vi "CreateTask.vi"(8 "error in":errorcluster, 10 "data":T1={"IMAQDeviceName"="", "LocalSavingPath"=path "", "Save"=enum."off", "Timeout"={"Value"=0.0, "Min"=0.0, "Max"=0.0, "StepSize"=0.0, "Tolerance"=0.0, "ValueActual"=0.0}, "Min Temperature"={"Value"=0.0, "Min"=18.0, "Max"=50.0, "StepSize"=0.0, "Tolerance"=0.0, "ValueActual"=0.0}, "aiChannel"="", "CJC_Value"={"Value"=0.0, "Min"=0.0, "Max"=0.0, "StepSize"=0.0, "Tolerance"=0.0, "ValueActual"=0.0}, "Thermocouple Type"=enum."E", "units"=enum."From Custom Scale", "CJC Source"=enum."Channel", "CJC Channel"="", "Simulation"=enum."off", "Max Temperature"={"Value"=0.0, "Min"=18.0, "Max"=50.0, "StepSize"=0.0, "Tolerance"=0.0, "ValueActual"=0.0}}, 11 "NI-TC-01 in":refnum<class "NI-TC-01.lvclass">) -> (0 "error out":errorcluster, 2 "data Out":T1={"IMAQDeviceName"="", "LocalSavingPath"=path "", "Save"=enum."off", "Timeout"={"Value"=0.0, "Min"=0.0, "Max"=0.0, "StepSize"=0.0, "Tolerance"=0.0, "ValueActual"=0.0}, "Min Temperature"={"Value"=0.0, "Min"=18.0, "Max"=50.0, "StepSize"=0.0, "Tolerance"=0.0, "ValueActual"=0.0}, "aiChannel"="", "CJC_Value"={"Value"=0.0, "Min"=0.0, "Max"=0.0, "StepSize"=0.0, "Tolerance"=0.0, "ValueActual"=0.0}, "Thermocouple Type"=enum."E", "units"=enum."From Custom Scale", "CJC Source"=enum."Channel", "CJC Channel"="", "Simulation"=enum."off", "Max Temperature"={"Value"=0.0, "Min"=18.0, "Max"=50.0, "StepSize"=0.0, "Tolerance"=0.0, "ValueActual"=0.0}}, 3 "NI-TC-01 out":refnum<class "NI-TC-01.lvclass">)   [LabVIEW 2013, in "NI-TC-01.lvclass"]
uses:
  NI-TC-01.lvclass
  settings_TypDef.ctl
  shared/OnOffTypeDef.ctl
  shared/numericVariable_TypeDef.ctl
  NI-TC-01.lvclass/NI-TC-01.ctl
  <vilib>/DAQmx/create/channels.llb/DAQmx Create Channel (AI-Temperature-Thermocouple).vi
  BaseDriver/BaseDriver.lvclass
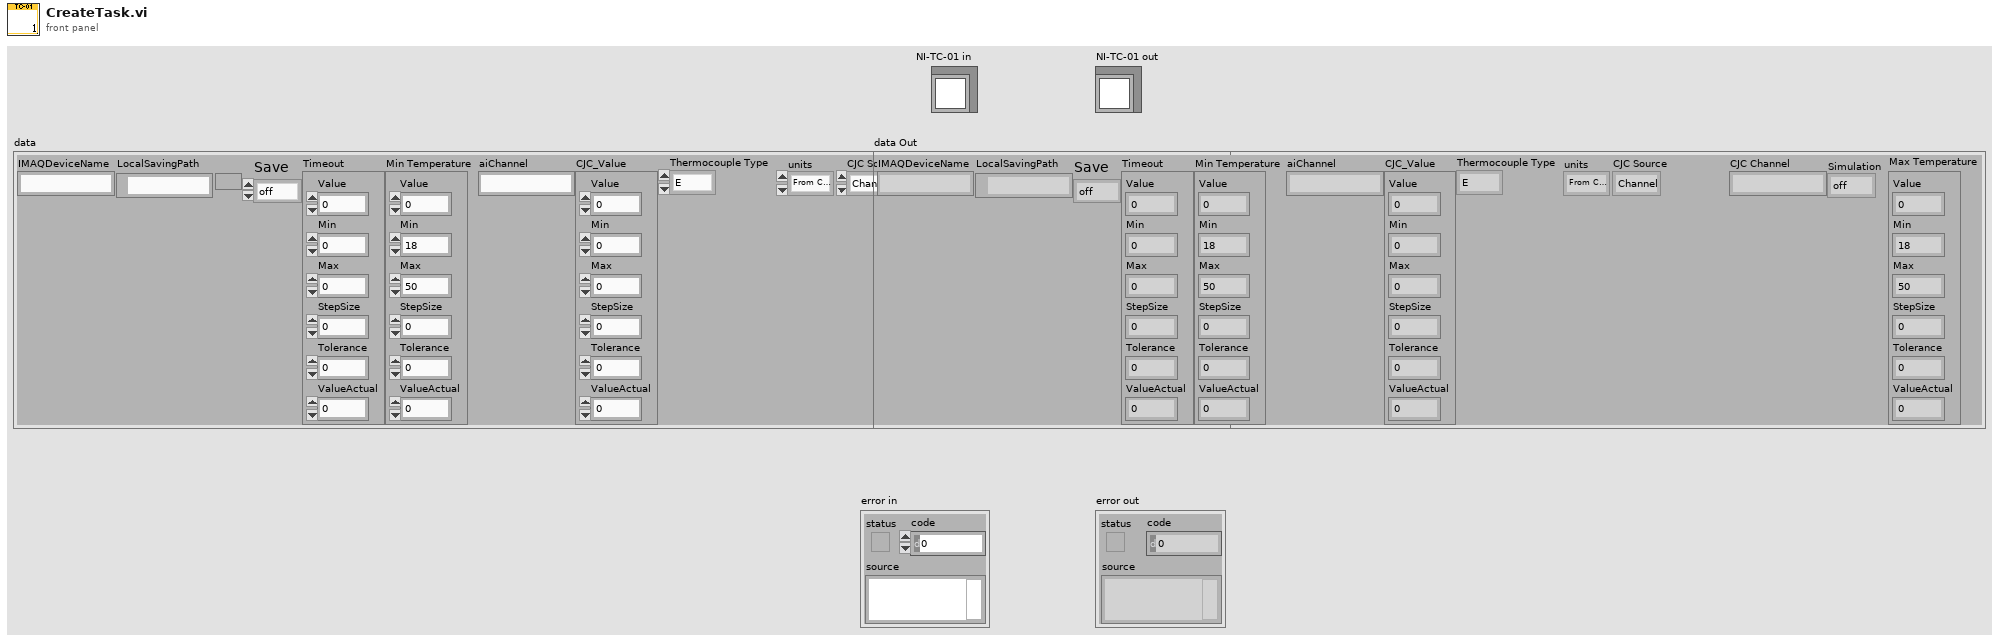
[diagram p1: front panel]
types:
  T1 = typedef "NI-TC-01.lvclass/settings_TypDef.ctl" = cluster{"IMAQDeviceName":string, "LocalSavingPath":path, "Save":T2, "Timeout":T3, "Min Temperature":T3, "aiChannel":string, "CJC_Value":T3, "Thermocouple Type":enum16{"J", "K", "N", "R", "S", "T", "B", "E"}, "units":enum16{"Deg C", "Deg F", "Kelvins", "Deg R", "From Custom Scale"}, "CJC Source":enum16{"Built-In", "Constant Value", "Channel"}, "CJC Channel":string, "Simulation":T2, "Max Temperature":T3}
  T2 = typedef "OnOffTypeDef.ctl" = enum16{"off", "on"}
  T3 = typedef "BaseDriver.lvclass/numericVariable_TypeDef.ctl" = cluster{"Value":dbl, "Min":dbl, "Max":dbl, "StepSize":dbl, "Tolerance":dbl, "ValueActual":dbl}
  T4 = enum16{"Deg C", "Deg F", "Kelvins", "Deg R", "From Custom Scale"}
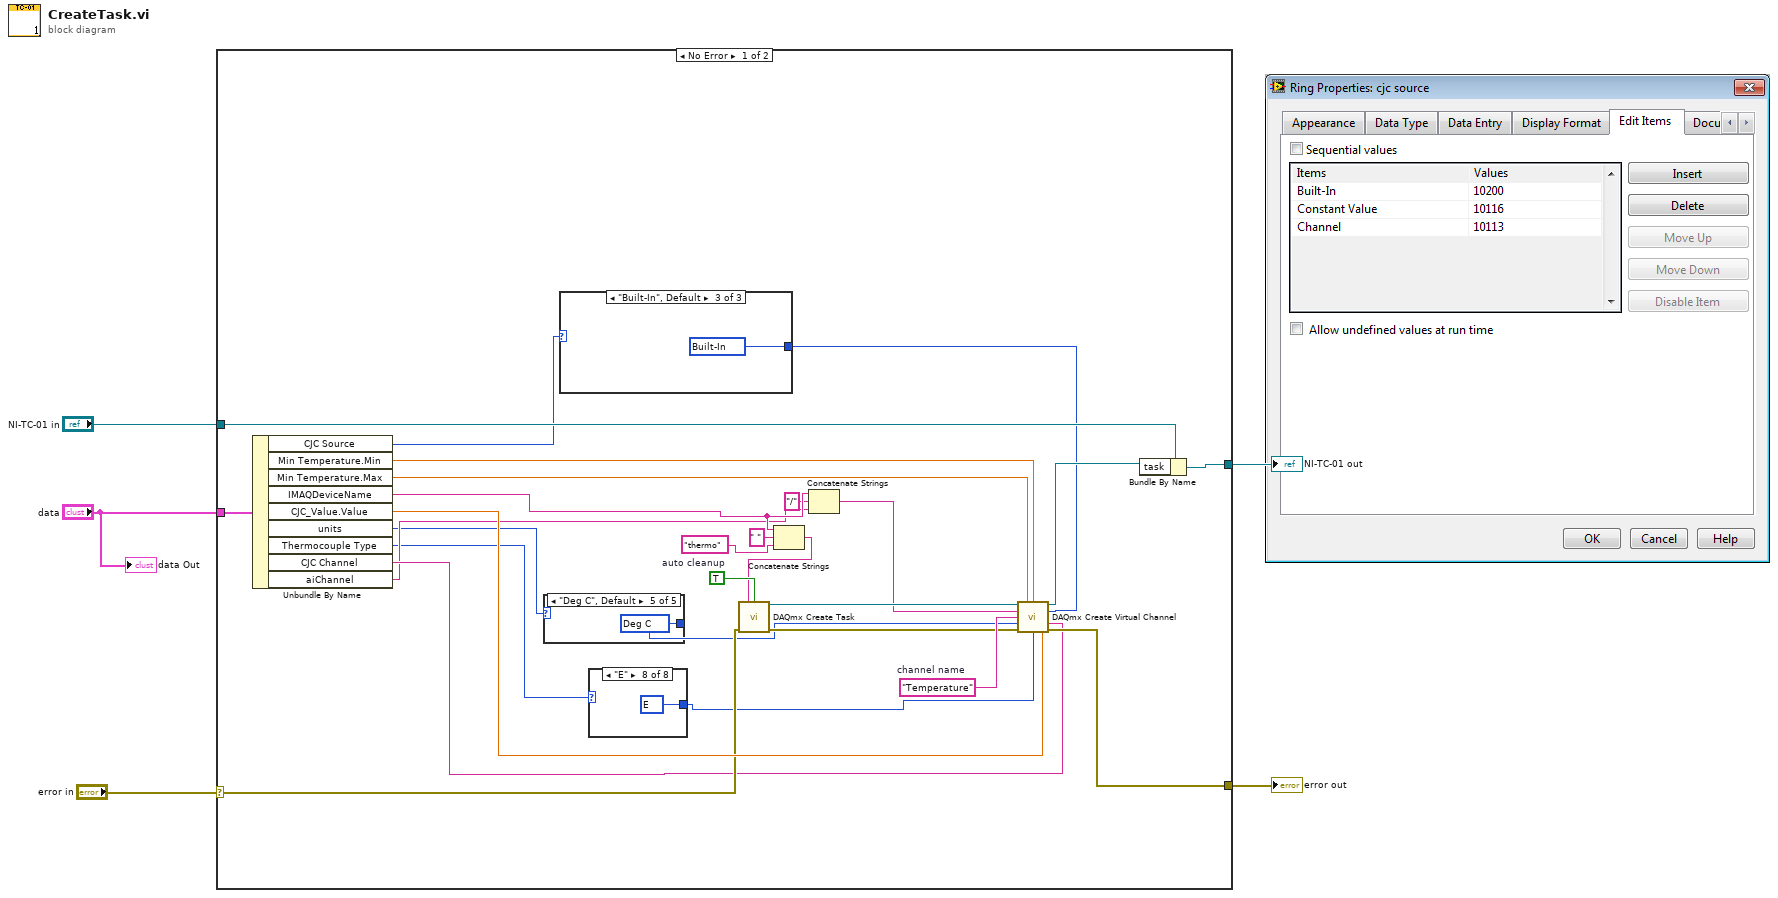
[diagram p0: block diagram]
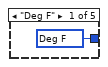
[diagram p2: hidden frame]
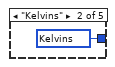
[diagram p3: hidden frame]
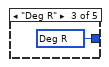
[diagram p4: hidden frame]
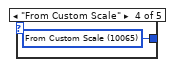
[diagram p5: hidden frame]
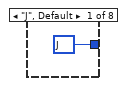
[diagram p6: hidden frame]
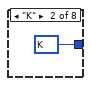
[diagram p7: hidden frame]
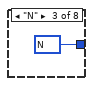
[diagram p8: hidden frame]
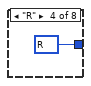
[diagram p9: hidden frame]
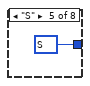
[diagram p10: hidden frame]
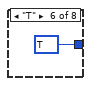
[diagram p11: hidden frame]
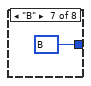
[diagram p12: hidden frame]
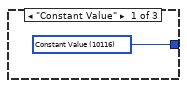
[diagram p13: hidden frame]
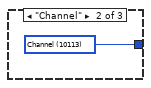
[diagram p14: hidden frame]
diagram:
  n1 = case shown="No Error" "error in" {
    selector: "error in" -> [w31 w50]
    tunnel: [w30 w50] -> w4
    tunnel: [w28 w49] -> w2
    tunnel: "NI-TC-01 in" -> [w29 w49]
    tunnel: "data" -> [w23 _]
    frame No Error {
      w21 = "Temperature"  # channel name
      w19 = TRUE  # auto cleanup
      n2 = Unbundle By Name(w23) -> ("CJC Source"=w11:enum16{"Built-In", "Constant Value", "Channel"}, "Min Temperature.Min"=w26:dbl, "Min Temperature.Max"=w25:dbl, "IMAQDeviceName"=w27:string, "CJC_Value.Value"=w32:dbl, "units"=w7:T4, "Thermocouple Type"=w9:enum16{"J", "K", "N", "R", "S", "T", "B", "E"}, "CJC Channel"=w24:string, "aiChannel"=w13:string)
      n3 = case shown="\"Deg C\", Default" w7 {
        tunnel: [w33 w34 w35 w36 w37] -> w6
        frame "Deg F" {
          w33 = 10144 items=["Deg C"=10143, "Deg F"=10144, "Kelvins"=10325, "Deg R"=10145, "From Custom Scale"=10065] ("units")
        }
        frame "Kelvins" {
          w34 = 10325 items=["Deg C"=10143, "Deg F"=10144, "Kelvins"=10325, "Deg R"=10145, "From Custom Scale"=10065] ("units")
        }
        frame "Deg R" {
          w35 = 10145 items=["Deg C"=10143, "Deg F"=10144, "Kelvins"=10325, "Deg R"=10145, "From Custom Scale"=10065] ("units")
        }
        frame "From Custom Scale" {
          w36 = 10065 items=["Deg C"=10143, "Deg F"=10144, "Kelvins"=10325, "Deg R"=10145, "From Custom Scale"=10065] ("units")
        }
        frame "Deg C", Default {
          w37 = 10143 items=["Deg C"=10143, "Deg F"=10144, "Kelvins"=10325, "Deg R"=10145, "From Custom Scale"=10065] ("units")
        }
      }
      n4 = case shown="\"Built-In\", Default" w11 {
        tunnel: [w46 w47 w48] -> w10
        frame "Constant Value" {
          w46 = 10116 items=["Built-In"=10200, "Constant Value"=10116, "Channel"=10113] ("cjc source")
        }
        frame "Channel" {
          w47 = 10113 items=["Built-In"=10200, "Constant Value"=10116, "Channel"=10113] ("cjc source")
        }
        frame "Built-In", Default {
          w48 = 10200 items=["Built-In"=10200, "Constant Value"=10116, "Channel"=10113] ("cjc source")
        }
      }
      n5 = case shown="\"E\"" w9 {
        tunnel: [w38 w39 w40 w41 w42 w43 w44 w45] -> w8
        frame "J", Default {
          w38 = 10072 items=["J"=10072, "K"=10073, "N"=10077, "R"=10082, "S"=10085, "T"=10086, "B"=10047, "E"=10055] ("thermocouple type")
        }
        frame "K" {
          w39 = 10073 items=["J"=10072, "K"=10073, "N"=10077, "R"=10082, "S"=10085, "T"=10086, "B"=10047, "E"=10055] ("thermocouple type")
        }
        frame "N" {
          w40 = 10077 items=["J"=10072, "K"=10073, "N"=10077, "R"=10082, "S"=10085, "T"=10086, "B"=10047, "E"=10055] ("thermocouple type")
        }
        frame "R" {
          w41 = 10082 items=["J"=10072, "K"=10073, "N"=10077, "R"=10082, "S"=10085, "T"=10086, "B"=10047, "E"=10055] ("thermocouple type")
        }
        frame "S" {
          w42 = 10085 items=["J"=10072, "K"=10073, "N"=10077, "R"=10082, "S"=10085, "T"=10086, "B"=10047, "E"=10055] ("thermocouple type")
        }
        frame "T" {
          w43 = 10086 items=["J"=10072, "K"=10073, "N"=10077, "R"=10082, "S"=10085, "T"=10086, "B"=10047, "E"=10055] ("thermocouple type")
        }
        frame "B" {
          w44 = 10047 items=["J"=10072, "K"=10073, "N"=10077, "R"=10082, "S"=10085, "T"=10086, "B"=10047, "E"=10055] ("thermocouple type")
        }
        frame "E" {
          w45 = 10055 items=["J"=10072, "K"=10073, "N"=10077, "R"=10082, "S"=10085, "T"=10086, "B"=10047, "E"=10055] ("thermocouple type")
        }
      }
      n6 = Concatenate Strings(w27, " " ("string"), "thermo" ("new task name")) -> (w14:string)
      n7 = call <vilib>:"DAQmx Create Task.vi"("new task name"=w14, "auto cleanup"=w19, "error in"=w31) -> ("task out"=w20:refnum<k21>, "error out"=w18:errorcluster)  [unwired: 11 in]
      n8 = Concatenate Strings(w27, "/" ("string"), w13) -> (w17:string)
      n9 = call-poly <vilib>:"DAQmx Create Virtual Channel.vi"("task in"=w20, "maximum value"=w25, "minimum value"=w26, "physical channels"=w17, "cjc source"=w10, "name to assign"=w21, "units"=w6, "cjc channel"=w24, "error in"=w18, "thermocouple type"=w8, "cjc value"=w32) -> ("task out"=w22:refnum<k21>, "error out"=w30:errorcluster)  [unwired: 3 in]
      n10 = Bundle By Name(cluster=w29, "task"=w22) -> (w28:refnum<class "NI-TC-01.lvclass">)
    }
    frame Error {
    }
  }
  "error out" <- w4
  "NI-TC-01 out" <- w2
  "data Out" <- "data"
